vi "Set_RAW.vi"(0 "reference in":refnum<class "Sig_Digital.lvclass">, 5 "RAW":bool, 11 "error in (no error)":errorcluster) -> (4 "reference out":refnum<class "Sig_Digital.lvclass">, 15 "error out":errorcluster)   [LabVIEW 2019, in "Sig_Digital.lvclass"]
uses:
  Sig_Digital.lvclass
  D:/H4000/src/Proccess_class/Proccess.lvclass
  Sig_Digital.lvclass/Sig_Digital.ctl
  Proccess_class/Proccess.lvclass/Proccess.ctl
  Proccess_class/Read TagName.vi
  Proccess_class/Read Logger.vi
  Logger_class/WriteEvent.vi
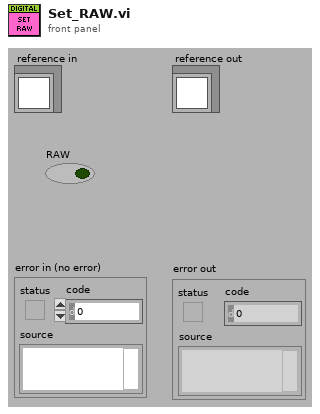
[diagram p1: front panel]
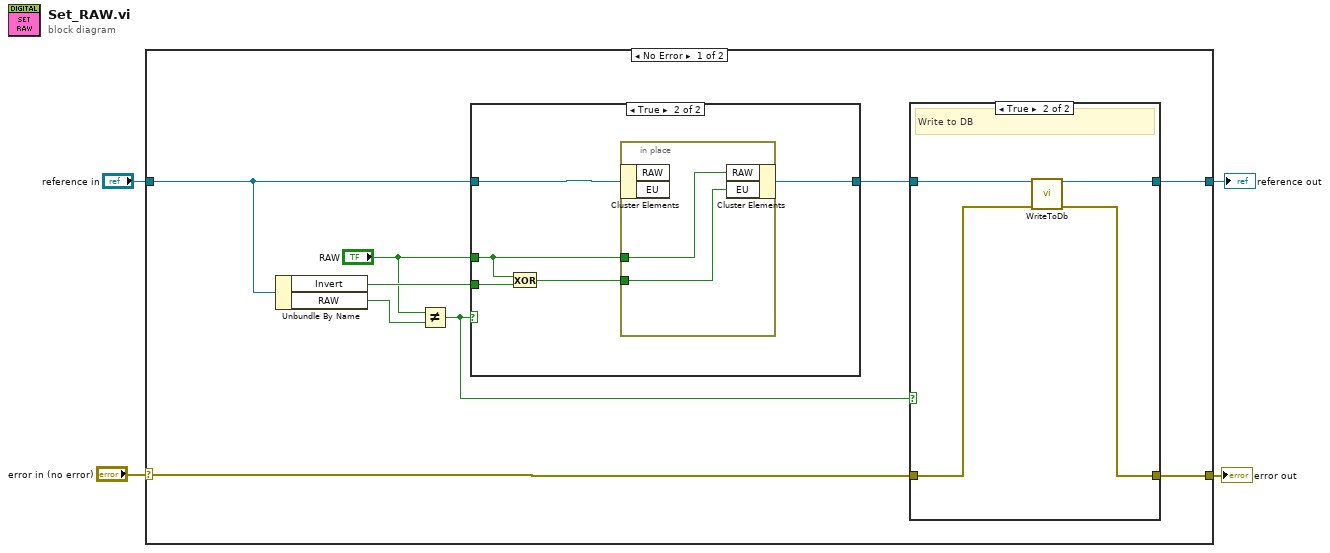
[diagram p0: block diagram]
diagram:
  n1 = case shown="No Error" "error in (no error)" {
    selector: "error in (no error)" -> [w13 w29]
    tunnel: [w7 w29] -> w3
    tunnel: [w9 w28] -> w1
    tunnel: "reference in" -> [w6 w28]
    frame No Error {
      n2 = Unbundle By Name(w6) -> ("Invert"=w12:bool, "RAW"=w10:bool)
      n3 = Not Equal?(x="RAW", y=w10) -> (x != y?=w8:bool)
      n4 = case shown="True" w8 {
        tunnel: w6 -> [w14 w16]
        tunnel: w12 -> [_ w19]
        tunnel: "RAW" -> [_ w17]
        tunnel: [w14 w15] -> w5
        frame False {
        }
        frame True {
          n5 = Exclusive Or(1:w19, 2:w17) -> (0:w18:bool)
          n6 = in-place {
            in-place-border: w17 -> [w21]
            in-place-border: w18 -> [w20]
            n7 = in-place-cluster #1(w16) -> ()  [unwired: 2 out]
            n8 = in-place-cluster #1("RAW"=w21, "EU"=w20) -> (w15:refnum<class "Sig_Digital.lvclass">)
          }
        }
      }
      n9 = case shown="True" w8 {
        tunnel: w5 -> [w23 w26]
        tunnel: [w23 w25] -> w9
        tunnel: w13 -> [w22 w27]
        tunnel: [w22 w24] -> w7
        frame False {
        }
        frame True {
          # "Write to DB"
          n10 = call "WriteToDb.vi"("reference in"=w26, "error in (no error)"=w27) -> ("reference out"=w25:refnum<class "Sig_Digital.lvclass">, "error out"=w24:errorcluster)  [unwired: 12 in]
        }
      }
    }
    frame Error {
    }
  }
  "error out" <- w3
  "reference out" <- w1
